vi "find_double_peaks_test.vi"() -> ()   [LabVIEW 2013]
uses:
  <vilib>/Utility/file.llb/Read From Spreadsheet File (DBL).vi
  Classes/Plots/Plots.lvclass
panel:
  in  "peak offset":dbl=0.00075
  out "XY Graph":cluster{cluster{dbl, "Numeric":dbl}[]}[](graph)
  out "fit coeff":T1
  in  "file path (dialog if empty)":path=path "C:/Users/Thermo/Documents/GitHub/HelixMC/MSControl/test_vis/double_peak_data.txt"
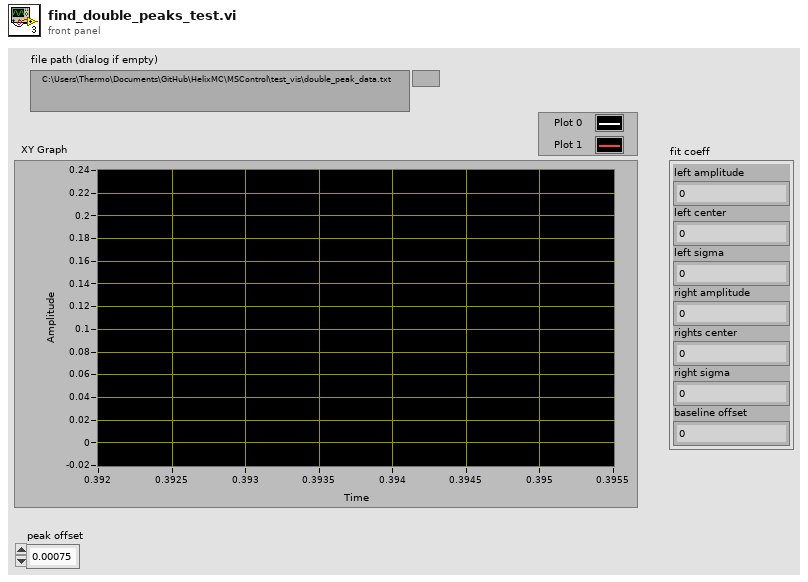
[diagram p1: front panel]
types:
  T1 = cluster{"left amplitude":dbl, "left center":dbl, "left sigma":dbl, "right amplitude":dbl, "rights center":dbl, "right sigma":dbl, "baseline offset":dbl}
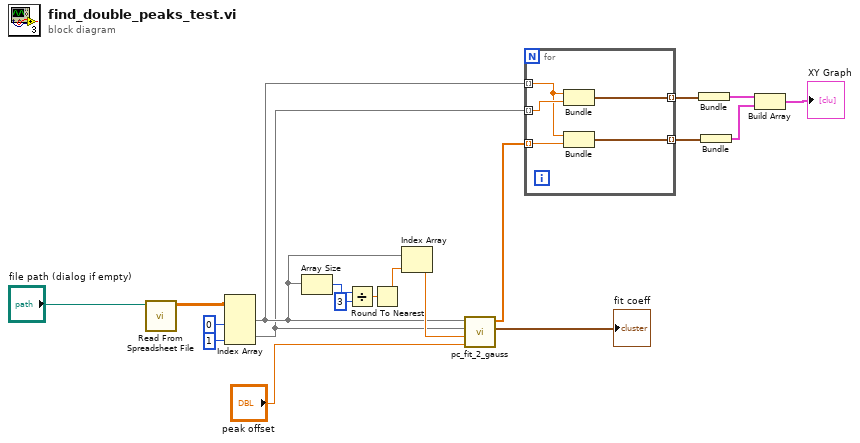
[diagram p0: block diagram]
diagram:
  n1 = call-poly <vilib>:"Read From Spreadsheet File.vi"("file path (dialog if empty)"="file path (dialog if empty)") -> ("all rows"=w10:dbl[][])  [unwired: 6 in, 4 out]
  n2 = Index Array(array=w10, index (col) #1=0 ("disabled index (col)"), index (col) #2=1 ("index (col)")) -> (element #1=w9:dbl[], element #2=w8:dbl[])  [unwired: 2 in]
  n3 = Array Size(array=w9) -> (size(s)=w12:i32)
  n4 = Divide(x=w12, y=3) -> (x/y=w14:dbl)
  n5 = Round To Nearest(number=w14) -> (nearest integer value=w15:dbl)
  n6 = Index Array(array=w9, index=w15) -> (element=w11:dbl)
  n7 = call "pc_fit_2_gauss.vi"("peak offset"="peak offset", "Center requested peak"=w11, "Y-Data"=w8, "X-Data"=w9) -> ("fit coeff"=→"fit coeff":T1, "best nonlinear fit"=w5:dbl[])  [unwired: 4 in, 2 out]
  n8 = for {
    tunnel: w9 -> [w22] mode=indexing
    tunnel: w8 -> [w24] mode=indexing
    tunnel: [w23] -> w7 mode=indexing
    tunnel: w5 -> [w21] mode=indexing
    tunnel: [w20] -> w4 mode=indexing
    n9 = Bundle(w22, w24) -> (w23:cluster{dbl, dbl})  [unwired: 1 in]
    n10 = Bundle(w22, "Numeric"=w21) -> (w20:cluster{dbl, "Numeric":dbl})  [unwired: 1 in]
  }
  n11 = Bundle(w7) -> (w6:cluster{cluster{dbl, dbl}[]})  [unwired: 1 in]
  n12 = Bundle(w4) -> (w3:cluster{cluster{dbl, "Numeric":dbl}[]})  [unwired: 1 in]
  n13 = Build Array(w6, w3) -> (→"XY Graph":cluster{cluster{dbl, "Numeric":dbl}[]}[])
